vi "Serial Test GB_TSFTS2_v2.vi"(8 "error in (no error)":errorcluster, 11 "ControlBoard VISA":refnum<visa-resource-name>="ControlBoard") -> (0 "error out":errorcluster, 2 "Message OUT":string, 3 "Result (bool)":bool)   [LabVIEW 2022 SP3]
uses:
  SupportVIs/VISA Flush IO Buffer Mask.ctl
panel:
  out "Expected Result":string
  out "Actual Result":string
  out "Result (color)":u32(colorbox)
  out "VISA resource OUT":refnum<visa-resource-name>
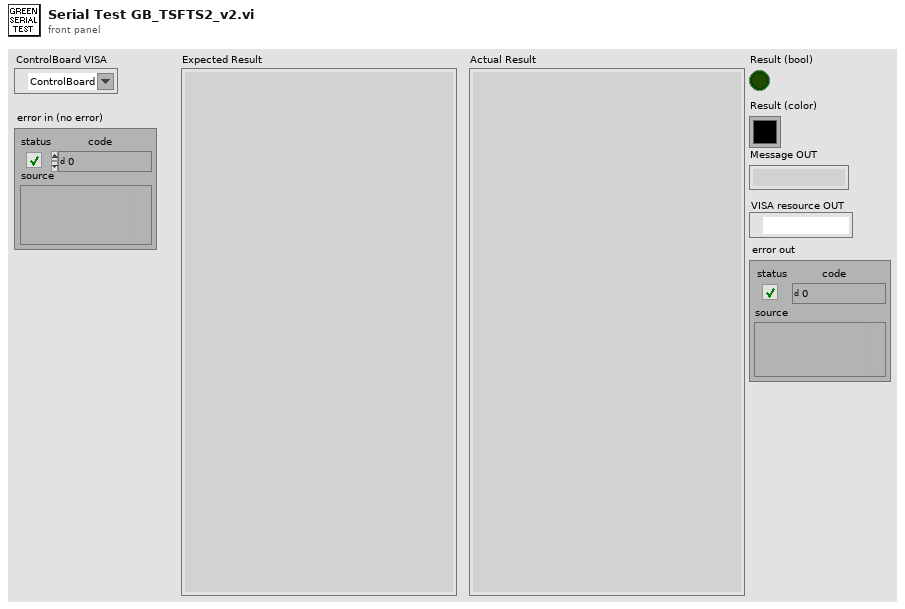
[diagram p1: front panel]
types:
  T1 = typedef "VISA Flush IO Buffer Mask.ctl" = u16
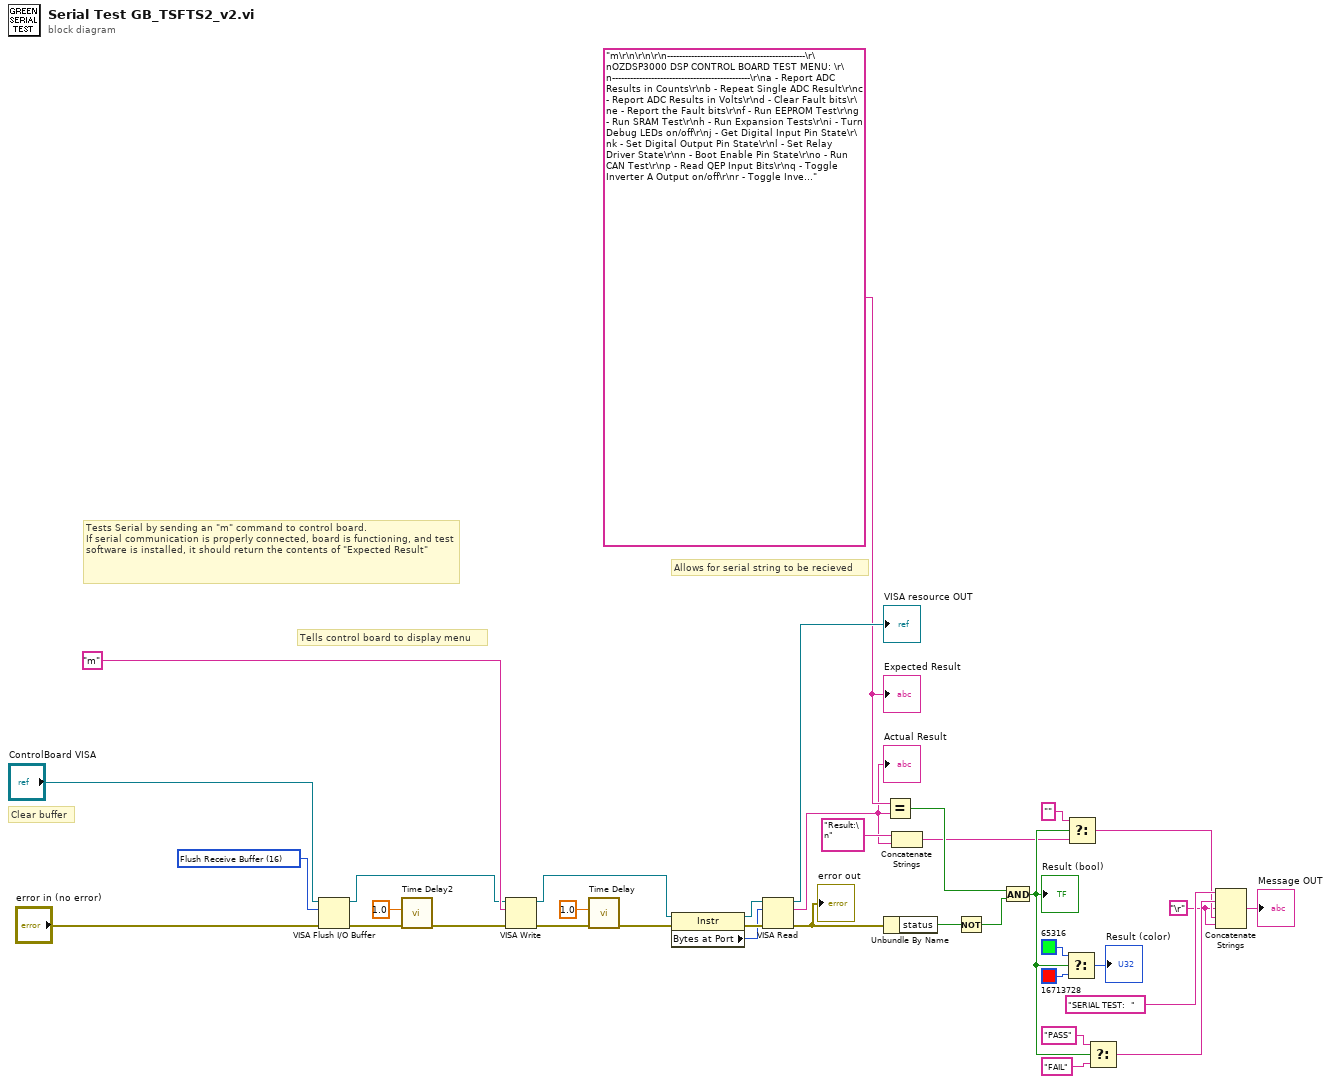
[diagram p0: block diagram]
diagram:
  w6 = "\r"
  w17 = "m\r\n\r\n\r\n----------------------------------------------\r\nOZDSP3000 DSP CONTROL BOARD TEST MENU: \r\n----------------------------------------------\r\na - Report ADC Results in Counts\r\nb - Repeat Single ADC Result\r\nc - Report ADC Results in Volts\r\nd - Clear Fault bits\r\ne - Report the Fault bits\r\nf - Run EEPROM Test\r\ng - Run SRAM Test\r\nh - Run Expansion Tests\r\ni - Turn Debug LEDs on/off\r\nj - Get Digital Input Pin State\r\nk - Set Digital Output Pin State\r\nl - Set Relay Driver State\r\nn - Boot Enable Pin State\r\no - Run CAN Test\r\np - Read QEP Input Bits\r\nq - Toggle Inverter A Output on/off\r\nr - Toggle Inverter B Output on/off\r\ns - Toggle Half Bridge Output on/off\r\nt - Set PWM leg duty cycle\r\nu - Real Time Clock\r\nv - Watchdog Control\r\nw - Test Interrupt Lines\r\nx - Read HALLs\r\ny - Test FPGA Read/Write\r\nz - Report Software/FPGA Revs\r\nm - Display this menu\r\n> "
  w32 = T1 16 items=["Flush Receive Buffer"=16, "Write Transmit Buffer to Device"=32, "Flush Receive Buffer (No I/O)"=64, "Flush Transmit Buffer"=128] ("Mask")
  # "Tests Serial by sending an \"m\" command to control board.\nIf serial communication is properly connected, board is functioning, and test software is installed, it should return the contents of \"Expected Result\""
  # "Clear buffer"
  # "Allows for serial string to be recieved"
  # "Tells control board to display menu"
  n1 = VISA Flush I/O Buffer(VISA resource name="ControlBoard VISA", mask (16)=w32, error in (no error)="error in (no error)") -> (VISA resource name out=w30:refnum<visa-resource-name>, error out=w5:errorcluster)
  n2 = call "Time Delay2"("error in (no error)"=w5, "Delay Time (s)"=1.0) -> ("error out"=w4:errorcluster)  [unwired: 9 in]
  n3 = VISA Write(VISA resource name=w30, write buffer="m", error in (no error)=w4) -> (VISA resource name out=w28:refnum<visa-resource-name>, error out=w31:errorcluster)  [unwired: 1 out]
  n4 = call "Time Delay"("error in (no error)"=w31, "Delay Time (s)"=1.0) -> ("error out"=w29:errorcluster)  [unwired: 9 in]
  n5 = property class="Instr"(reference=w28, error in=w29) -> (reference out=w35:refnum<visa-resource-name>, error out=w34:errorcluster, "Bytes at Port"=w33:u32)
  n6 = VISA Read(VISA resource name=w35, byte count=w33, error in (no error)=w34) -> (VISA resource name out=→"VISA resource OUT":refnum<visa-resource-name>, read buffer=w11:string, error out=w18:errorcluster)  [unwired: 1 out]
  "error out" <- w18
  "Actual Result" <- w11
  n7 = Unbundle By Name(w18) -> ("status"=w25:bool)
  n8 = Equal?(x=w17, y=w11) -> (x = y?=w19:bool)
  n9 = Concatenate Strings("Result:\n", w11) -> (w8:string)
  n10 = Not(x=w25) -> (.not. x?=w26:bool)
  n11 = And(x=w19, y=w26) -> (x .and. y?=w10:bool)
  "Result (bool)" <- w10
  n12 = Select(t=u32 65316 ("Result (color)"), s=w10, f=u32 16713728 ("Result (color)")) -> (s? t:f=→"Result (color)":u32)
  n13 = Select(t="", s=w10, f=w8) -> (s? t:f=w9:string)
  n14 = Select(t="PASS", s=w10, f="FAIL") -> (s? t:f=w13:string)
  n15 = Concatenate Strings("SERIAL TEST:  ", w13, w6, w9, w6) -> (→"Message OUT":string)
  "Expected Result" <- w17
